vi "Galil_DR.vi"() -> ()   [LabVIEW 2011]
panel:
  in  "Galil.IGalil":refnum<k7>
  out "DR event error":errorcluster
  out "OFFLINE error":errorcluster
  out "TIME":dbl
  in  "stop":bool
  in  "record":variant
  out "Library Version:":string
  out "error out":errorcluster
  out "Descrption":string[](array[string])
  out "Units":string[](array[string])
  out "sourceValue":dbl[](array[numeric])
  out "Number of Elements\nin Data Record":i32
  out "Sources":string[](array[string])
  out "For error out":errorcluster
  out "Connected To:":string
  in  "Connection String:":string
  # "This vi shows how to access data record information using the DR method (onRecord event) with the Galil Communications Library.  \n\nIf Connection String is left blank, the vi will open the connections dialog when run.  If a value is input into Connection String, the vi will attempt to connect to the controller at that address (ex COM1 19200).\n\nThis vi gets the full data record and constantatly updates the sourceValue, Units and Description arrays until the stop button is pressed.  This vi uses the DR method for obtaining the data record information.  The data record is sent out at a set interval from the controller, and the event_record.vi handles the onRecord event and passes the data to the Galil_DR.vi and displays it in the arrays shown for sourceValue, Units and Description.\n\nThe vi will run until the STOP button is pressed.  The STOP button should be used to stop the VI."
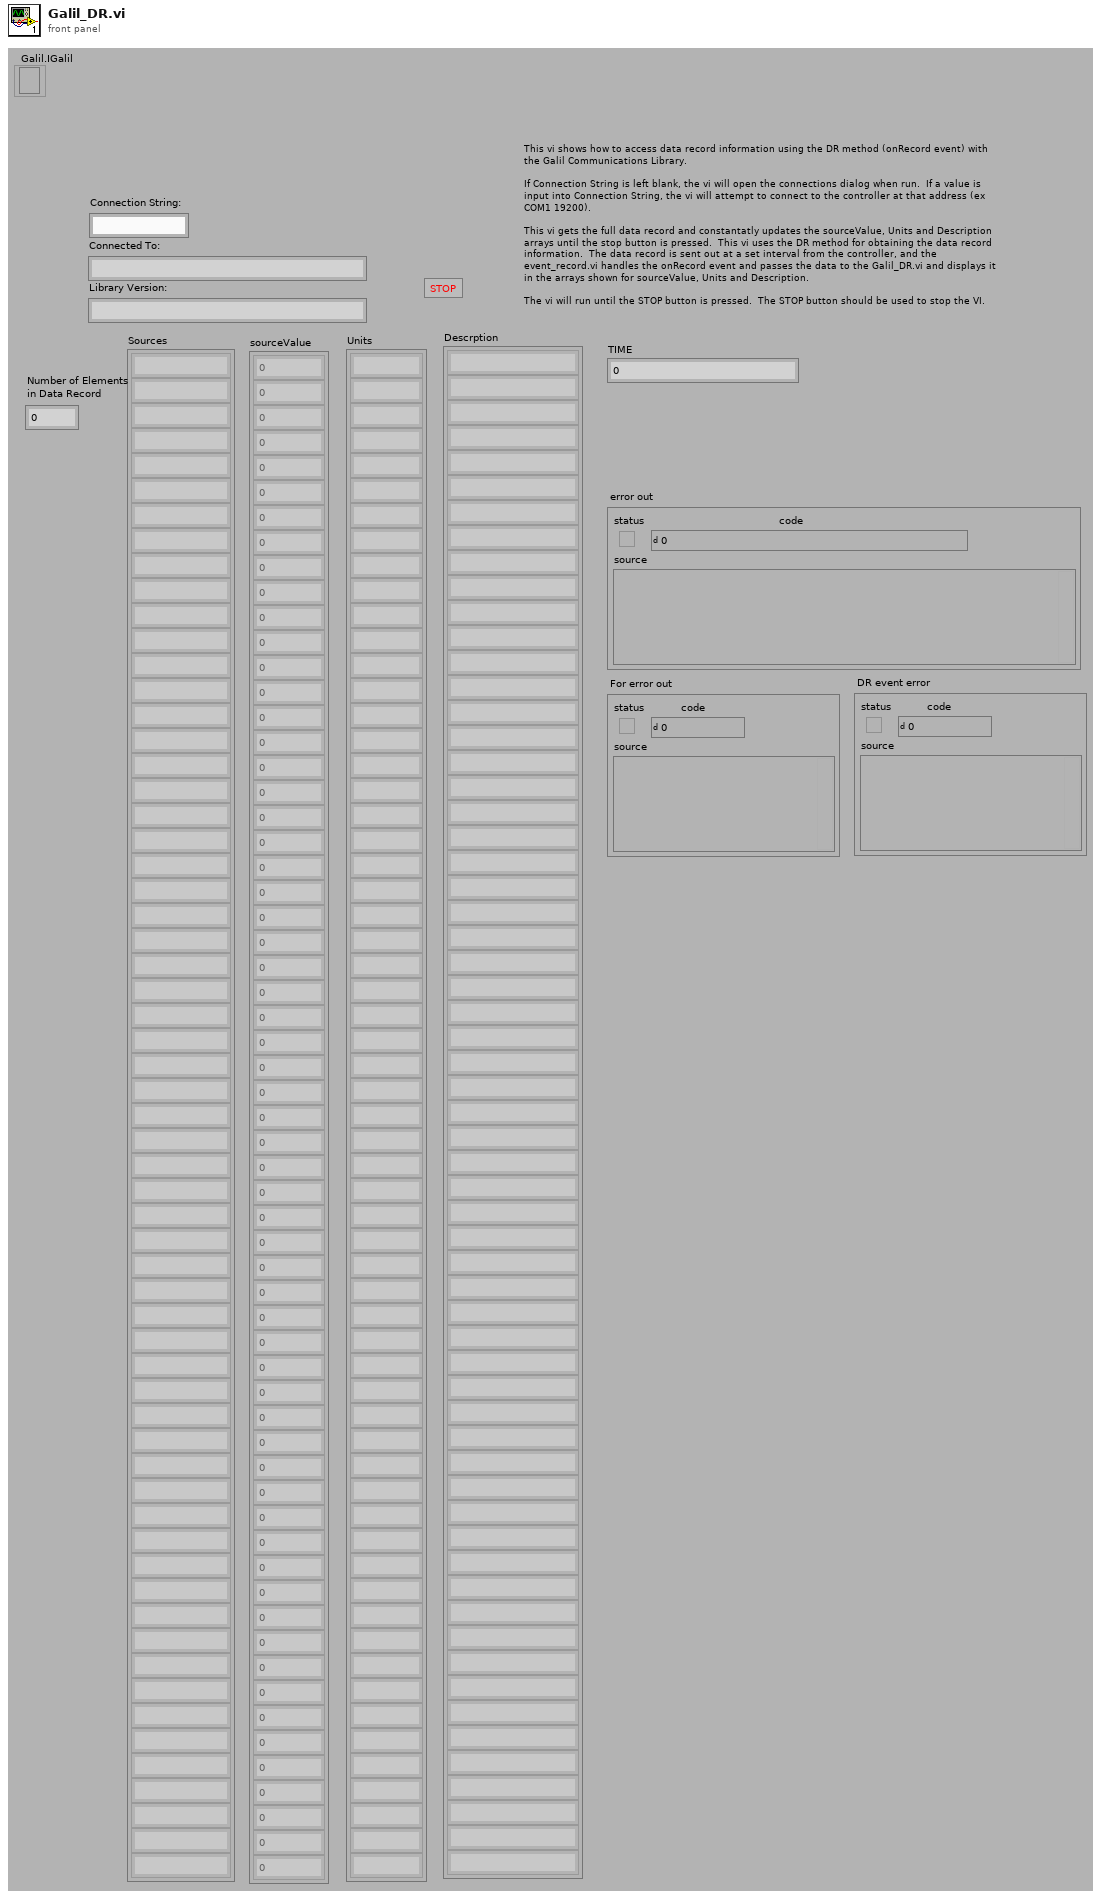
[diagram p1: front panel]
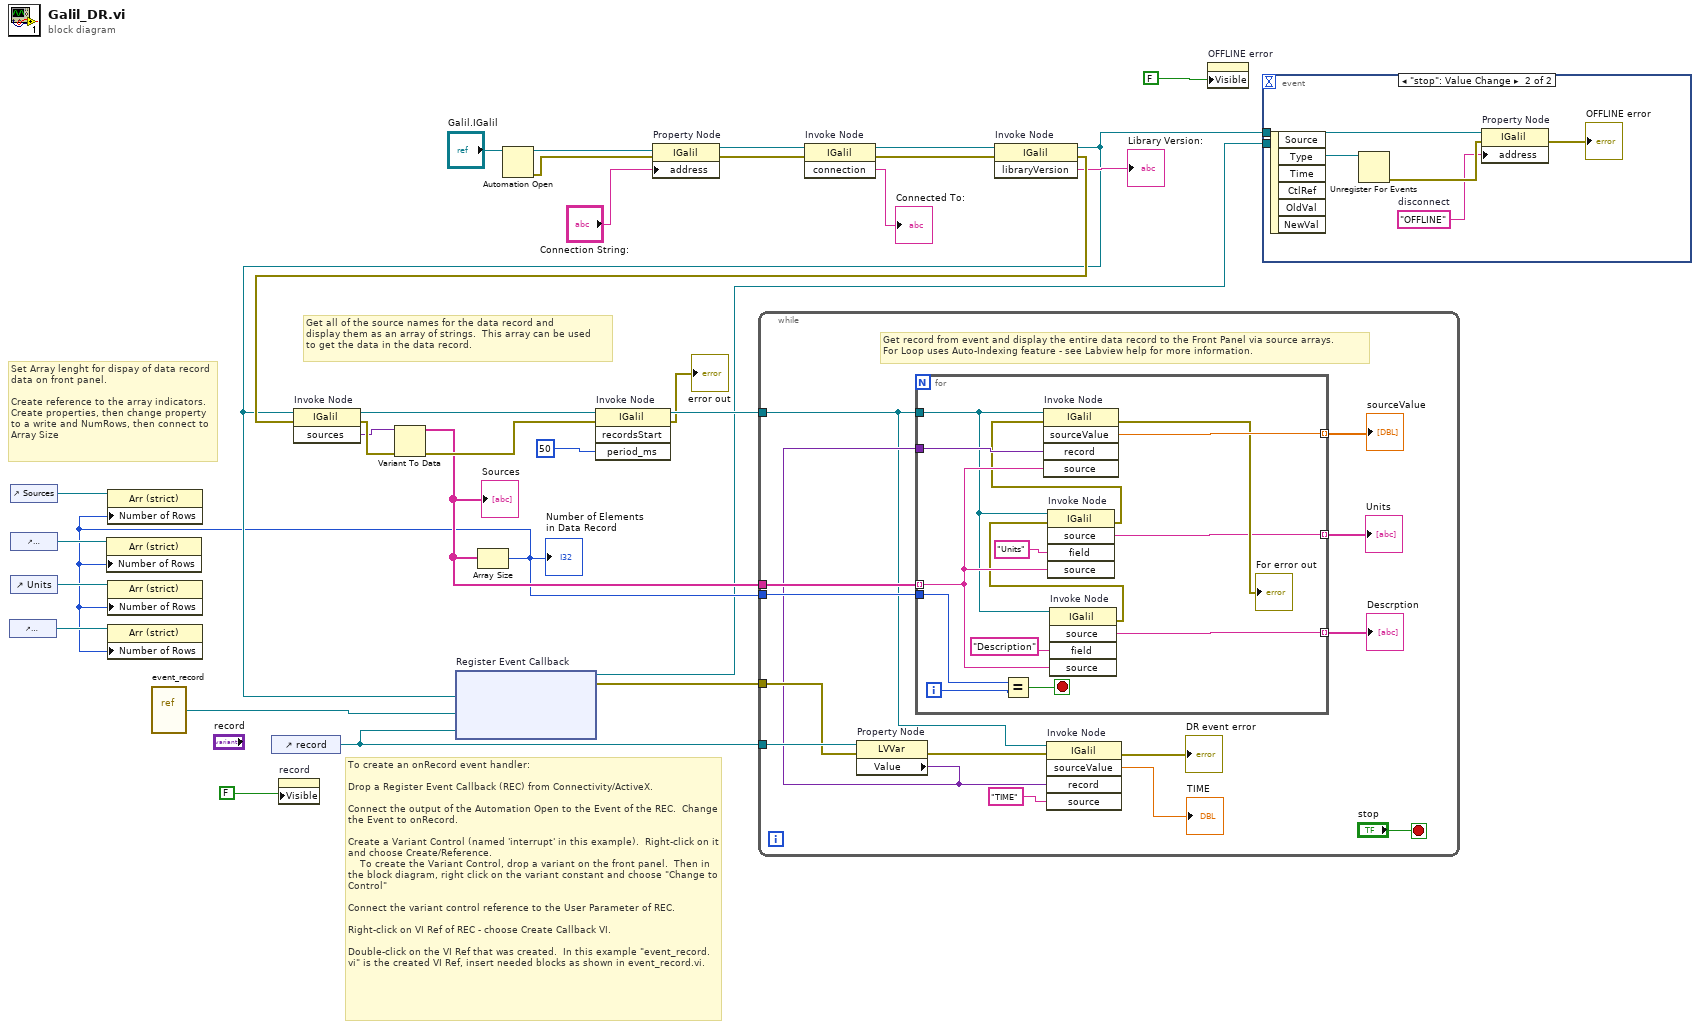
[diagram p0: block diagram]
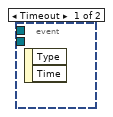
[diagram p2: hidden frame]
diagram:
  # "To create an onRecord event handler:\n\nDrop a Register Event Callback (REC) from Connectivity/ActiveX.  \n\nConnect the output of the Automation Open to the Event of the REC.  Change the Event to onRecord.\n\nCreate a Variant Control (named 'interrupt' in this example).  Right-click on it and choose Create/Reference. \n    To create the Variant Control, drop a variant on the front panel.  Then in the block diagram, right click on the variant constant and choose \"Change to Control\"\n\nConnect the variant control reference to the User Parameter of REC.\n\nRight-click on VI Ref of REC - choose Create Callback VI. \n\nDouble-click on the VI Ref that was created.  In this example \"event_record.vi\" is the created VI Ref, insert needed blocks as shown in event_record.vi."
  # "Set Array lenght for dispay of data record \ndata on front panel.\n\nCreate reference to the array indicators.  Create properties, then change property to a write and NumRows, then connect to Array Size"
  # "Get all of the source names for the data record and \ndisplay them as an array of strings.  This array can be used\nto get the data in the data record."
  n1 = control-ref of="Descrption"() -> (w15:refnum<vi>)
  n2 = control-ref of="Sources"() -> (w18:refnum<vi>)
  n3 = control-ref of="sourceValue"() -> (w17:refnum<vi>)
  n4 = control-ref of="Units"() -> (w16:refnum<vi>)
  n5 = vi-ref "event_record.vi"() -> ("vi reference"=w12:refnum<vi>)
  n6 = control-ref of="record"() -> (w10:refnum<vi>)
  n7 = property on="record" class="LVVar"("Visible"=FALSE) -> ()  [unwired: 2 in, 2 out]
  n8 = Automation Open(Automation Refnum="Galil.IGalil") -> (Automation Refnum=w14:refnum<k7>, error out=w30:errorcluster)  [unwired: 1 in, 2 out]
  n9 = property on="Property Node" class="IGalil"(reference=w14, error in=w30, "address"="Connection String:") -> (reference out=w31:refnum<k7>, error out=w29:errorcluster)
  n10 = invoke on="Invoke Node" class="IGalil" method="connection"(reference=w31, error in=w29) -> (reference out=w25:refnum<k7>, error out=w24:errorcluster, "connection"=→"Connected To:":string)  [unwired: 1 in]
  n11 = invoke on="Invoke Node" class="IGalil" method="libraryVersion"(reference=w25, error in=w24) -> (reference out=w11:refnum<k7>, error out=w23:errorcluster, "libraryVersion"=→"Library Version:":string)  [unwired: 1 in]
  n12 = invoke on="Invoke Node" class="IGalil" method="sources"(reference=w11, error in=w23) -> (reference out=w20:refnum<k7>, error out=w26:errorcluster, "sources"=w13:variant)  [unwired: 1 in]
  n13 = Variant To Data(error in=w26, Variant=w13) -> (data=w7:string[], error out=w19:errorcluster)  [unwired: 1 in]
  "Sources" <- w7
  n14 = node "Register Event Callback"(w11, w12, w10) -> (w5:refnum<k27>, w9:errorcluster)  [unwired: 2 in]
  n15 = Array Size(array=w7) -> (size(s)=w6:i32)
  "Number of Elements\nin Data Record" <- w6
  n16 = property class="Arr (strict)"(reference=w17, "Number of Rows"=w6) -> ()  [unwired: 1 in, 2 out]
  n17 = property class="Arr (strict)"(reference=w18, "Number of Rows"=w6) -> ()  [unwired: 1 in, 2 out]
  n18 = property class="Arr (strict)"(reference=w16, "Number of Rows"=w6) -> ()  [unwired: 1 in, 2 out]
  n19 = property class="Arr (strict)"(reference=w15, "Number of Rows"=w6) -> ()  [unwired: 1 in, 2 out]
  n20 = invoke on="Invoke Node" class="IGalil" method="recordsStart"(reference=w20, error in=w19, "period_ms"=50) -> (reference out=w8:refnum<k7>, error out=→"error out":errorcluster)  [unwired: 1 in, 2 out]
  n21 = while {
    tunnel: w10 -> [w40]
    tunnel: w9 -> [w36]
    tunnel: w8 -> [w34]
    tunnel: w7 -> [w39]
    tunnel: w6 -> [w38]
    stop <- "stop" stop-if-true
    # "Get record from event and display the entire data record to the Front Panel via source arrays.\nFor Loop uses Auto-Indexing feature - see Labview help for more information."
    n22 = property on="Property Node" class="LVVar"(reference=w40, error in=w36) -> (error out=w41:errorcluster, "Value"=w35:variant)  [unwired: 1 out]
    n23 = for {
      tunnel: [w58] -> w37 mode=indexing
      tunnel: w34 -> [w48]
      tunnel: w38 -> [w56]
      tunnel: w39 -> [w51] mode=indexing
      tunnel: w35 -> [w55]
      tunnel: [w52] -> w33 mode=indexing
      tunnel: [w49] -> w32 mode=indexing
      i -> [w57]
      stop <- w59 stop-if-true
      n24 = Equal?(x=w56, y=w57) -> (x = y?=w59:bool)
      n25 = invoke on="Invoke Node" class="IGalil" method="source"(reference=w48, "field"="Description", "source"=w51) -> (error out=w47:errorcluster, "source"=w49:string)  [unwired: 2 in, 3 out]
      n26 = invoke on="Invoke Node" class="IGalil" method="source"(reference=w48, error in=w47, "field"="Units", "source"=w51) -> (error out=w46:errorcluster, "source"=w52:string)  [unwired: 1 in, 3 out]
      n27 = invoke on="Invoke Node" class="IGalil" method="sourceValue"(reference=w48, error in=w46, "record"=w55, "source"=w51) -> (error out=→"For error out":errorcluster, "sourceValue"=w58:dbl)  [unwired: 1 in, 3 out]
    }
    "sourceValue" <- w37
    "Units" <- w33
    "Descrption" <- w32
    n28 = invoke on="Invoke Node" class="IGalil" method="sourceValue"(reference=w34, error in=w41, "record"=w35, "source"="TIME") -> (error out=→"DR event error":errorcluster, "sourceValue"=→"TIME":dbl)  [unwired: 1 in, 3 out]
  }
  n29 = property on="OFFLINE error" class="Clust (strict)"("Visible"=FALSE) -> ()  [unwired: 2 in, 2 out]
  n30 = event shown="[1] \"stop\": Value Change" {
    selector: _ -> [_ _]
    dyn-events: _ -> [_ _]
    timeout: _ -> [_ _]
    tunnel: w11 -> [_ w61]
    tunnel: w5 -> [_ w60]
    event Timeout {
      n31 = event-data() -> ()  [unwired: 3 out]
    }
    event "stop": Value Change {
      w62 = "OFFLINE"  # disconnect
      n32 = event-data() -> ()  [unwired: 7 out]
      n33 = Unregister For Events(event registration refnum=w60) -> (error out=w63:errorcluster)  [unwired: 1 in]
      n34 = property on="Property Node" class="IGalil"(reference=w61, error in=w63, "address"=w62) -> (error out=→"OFFLINE error":errorcluster)  [unwired: 1 out]
    }
  }
